vi "SendThread.vi"() -> ()   [LabVIEW 2011]
uses:
  VIs/_USB_CAN_T_R_Unit_.ctl
  VIs/_USB_CAN_GLOBAL_.vi
panel:
  in  "channels":i32=2
  in  "TFun":u16
  in  "DeviceInd":u32
  in  "channel":u16(ring) items=["通道0", "通道1"]
  in  "type":u16(ring)=2 items=["USB-CAN"=2, "USB-CAN2.0"=3]
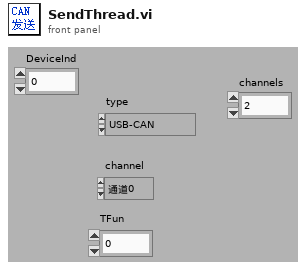
[diagram p1: front panel]
types:
  T1 = typedef "_USB_CAN_T_R_Unit_.ctl" = cluster{"time":timestamp, "channel":u16, "TimeStamp":u32, "tr":enum16{"接收", "发送"}, "id":u32, "Type":enum16{"数据帧", "远程帧"}, "Format":enum16{"标准帧", "扩展帧"}, "len":u8, "data":u8[]}
  T2 = typedef "_USB_CAN_SEND_BUFF_UNIT_.ctl" = cluster{"datalen":u8, "data":u8[], "id":u8[], "extended":bool, "remote":bool}
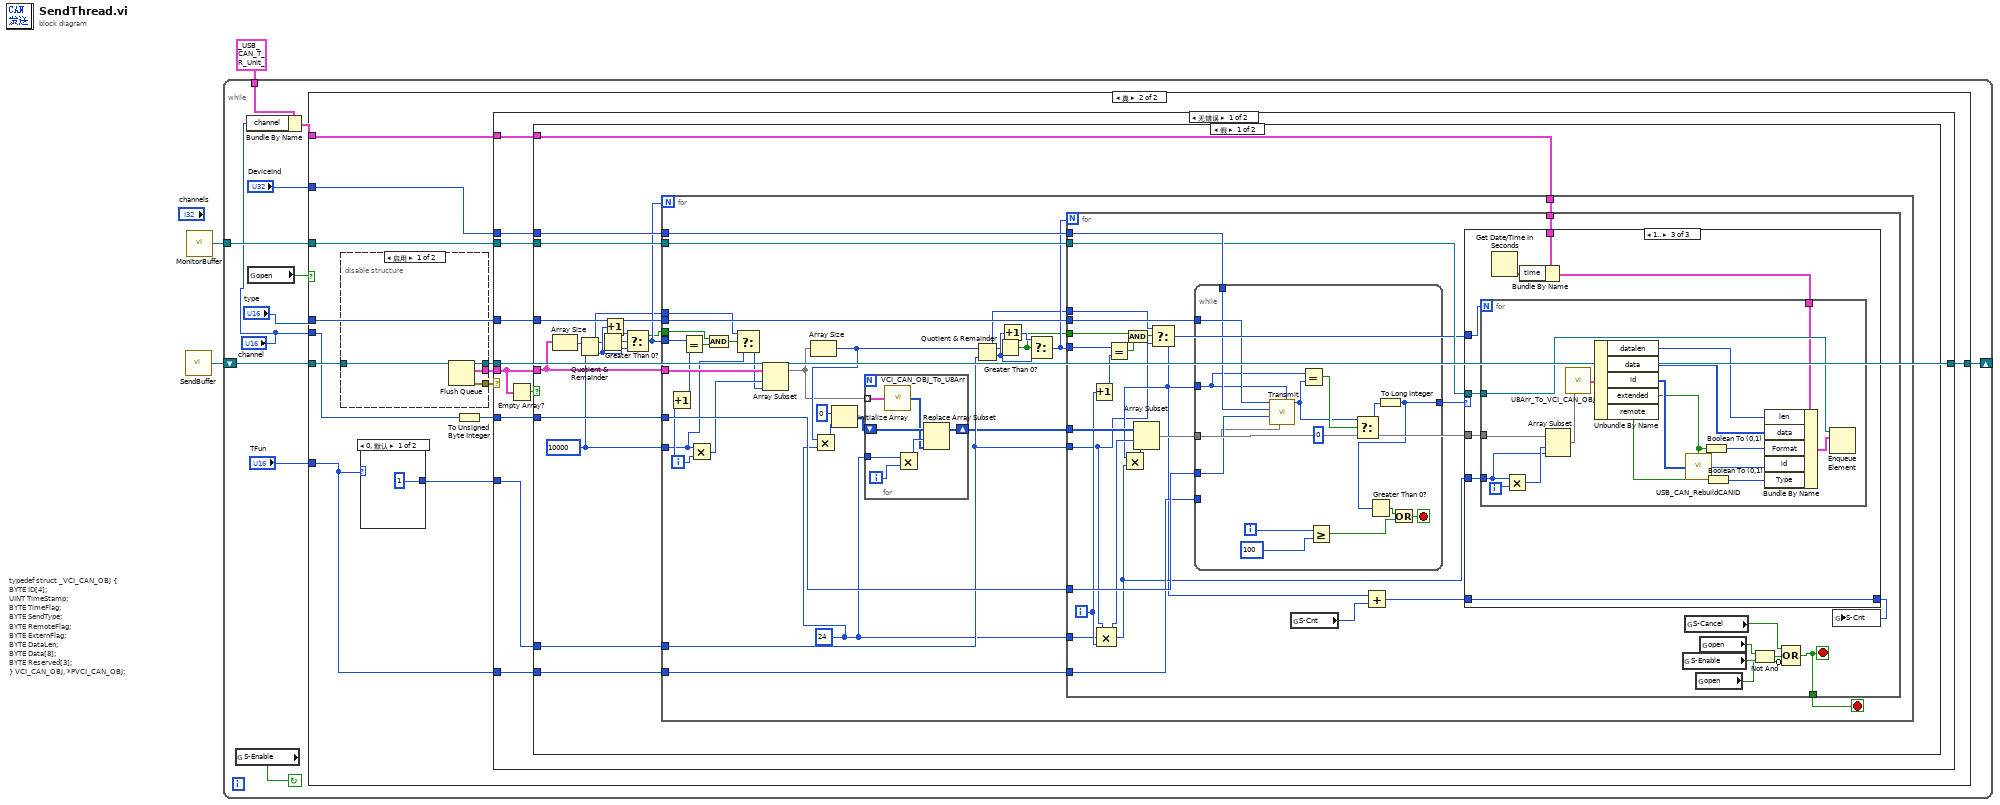
[diagram p0: block diagram]
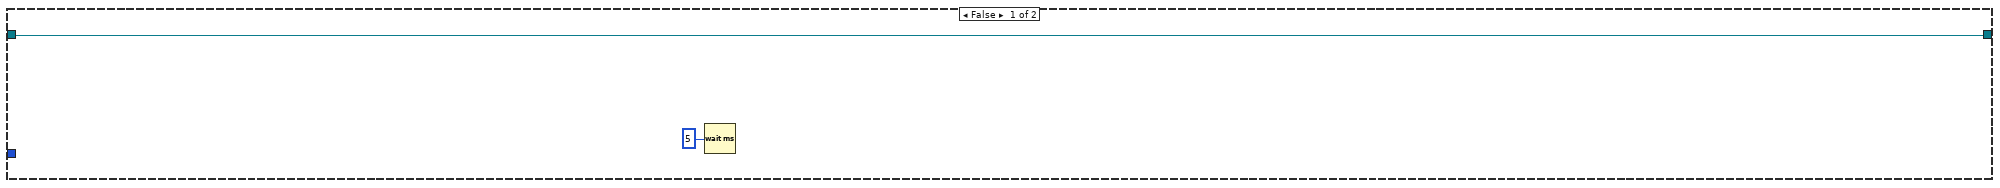
[diagram p2: hidden frame]
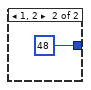
[diagram p3: hidden frame]
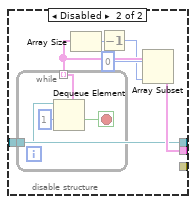
[diagram p4: hidden frame]
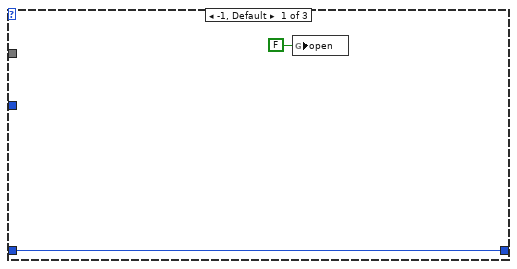
[diagram p5: hidden frame]
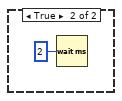
[diagram p7: hidden frame]
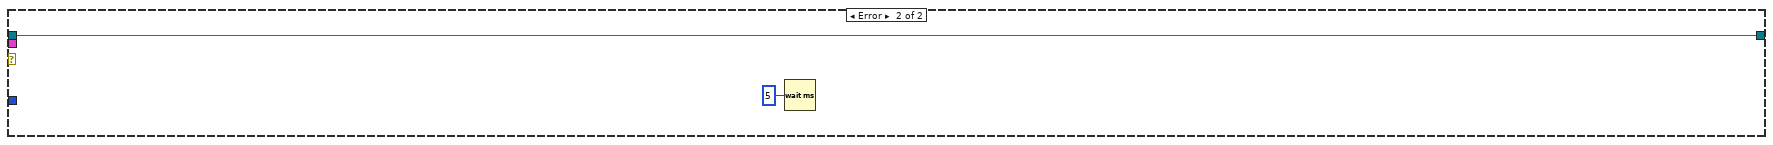
[diagram p8: hidden frame]
diagram:
  # "typedef struct _VCI_CAN_OBJ { \nBYTE ID[4];\nUINT TimeStamp; \nBYTE TimeFlag;\nBYTE SendType; \nBYTE RemoteFlag; \nBYTE ExternFlag; \nBYTE DataLen; \nBYTE Data[8]; \nBYTE Reserved[3];\n} VCI_CAN_OBJ, *PVCI_CAN_OBJ;"
  n1 = call "SendBuffer.vi"() -> ("VCI_CAN_BUF_T"=w3:refnum<queue>)  [unwired: 1 in]
  n2 = call "MonitorBuffer.vi"() -> ("USB_CAN_M_BUF"=w2:refnum<queue>)  [unwired: 1 in]
  n3 = while {
    shift-right: [w13] -> _
    shift-left: w3 -> [w14]
    tunnel: w2 -> [w8]
    tunnel: T1 {"time"=timestamp(0 s since 1904-01-01), "channel"=0, "TimeStamp"=0, "tr"=enum."发送", "id"=0, "Type"=enum."数据帧", "Format"=enum."标准帧", "len"=0, "data"=[]} ("元素") -> [w7]
    stop <- w12 continue-if-true
    n4 = global read "_USB_CAN_GLOBAL_.vi" "S-Enable"() -> (w12:bool)
    n5 = Bundle By Name(cluster=w7, "channel"="channel") -> (w5:T1)
    n6 = global read "_USB_CAN_GLOBAL_.vi" "open"() -> (w11:bool)
    n7 = case shown="真" w11 {
      tunnel: "type" -> [_ w25]
      tunnel: "channel" -> [_ w24]
      tunnel: w14 -> [w16 w29]
      tunnel: [w16 w26] -> w13
      tunnel: w8 -> [_ w22]
      tunnel: "DeviceInd" -> [_ w21]
      tunnel: "TFun" -> [_ w18]
      tunnel: w5 -> [_ w19]
      frame False {
        n8 = Wait (ms)(milliseconds to wait=u32 5 ("millisecond multiple")) -> ()  [unwired: 1 out]
      }
      frame True {
        n9 = disable-structure shown="启用" {
          disable-tunnel: w29 -> [w35 w36]
          disable-tunnel: [w34 _] -> w28
          disable-tunnel: [w33 w36] -> w27
          disable-tunnel: [w32 w37] -> w20
          frame Enabled {
            n10 = Flush Queue(queue=w35) -> (queue out=w33:refnum<queue>, remaining elements=w32:T2[], error out=w34:errorcluster)  [unwired: 1 in]
          }
          frame Disabled {
            n11 = while {
              tunnel: w36 -> [w45]
              tunnel: [w43] -> w40 mode=indexing
              stop <- w42 stop-if-true
              n12 = Dequeue Element(queue=w45, timeout in ms (-1)=1 ("超时毫秒(-1)")) -> (element=w43:T2, timed out?=w42:bool)  [unwired: 1 in, 2 out]
            }
            n13 = Array Size(array=w40) -> (size(s)=w41:i32)
            n14 = Decrement(x=w41) -> (x-1=w38:i32)
            n15 = Array Subset(array=w40, index=0 ("索引"), length=w38) -> (w37:T2[])
          }
        }
        n16 = case shown="0, 默认" w18 {
          tunnel: [1 ("索引") 48 ("索引")] -> w17
          frame 0, Default {
          }
          frame 1, 2 {
          }
        }
        n17 = To Unsigned Byte Integer(number=w24) -> (unsigned 8bit integer=w23:u8)
        n18 = case shown="无错误" w28 {
          tunnel: w27 -> [w50 w184]
          tunnel: [w50 w184] -> w26
          tunnel: w20 -> [w48 _]
          tunnel: w25 -> [w51 _]
          tunnel: w23 -> [w54 _]
          tunnel: w22 -> [w49 _]
          tunnel: w21 -> [w55 _]
          tunnel: w17 -> [w53 _]
          tunnel: w18 -> [w52 _]
          tunnel: w19 -> [w46 _]
          frame No Error {
            n19 = Empty Array?(array=w48) -> (empty?=w47:bool)
            n20 = case shown="假" w47 {
              tunnel: w55 -> [w70 _]
              tunnel: w54 -> [w69 _]
              tunnel: w53 -> [w65 _]
              tunnel: w52 -> [w68 _]
              tunnel: w51 -> [w67 _]
              tunnel: w49 -> [w66 _]
              tunnel: w48 -> [w63 _]
              tunnel: w46 -> [w64 _]
              frame False {
                w59 = 10000 ("y")
                n21 = Array Size(array=w63) -> (size(s)=w62:i32)
                n22 = Quotient & Remainder(x=w62, y=w59) -> (x-y*floor(x/y)=w56:i32, floor(x/y)=w60:i32)
                n23 = Greater Than 0?(x=w56) -> (x > 0?=w57:bool)
                n24 = Increment(x=w60) -> (x+1=w61:i32)
                n25 = Select(t=w61, s=w57, f=w60) -> (s? t:f=w58:i32)
                n26 = for {
                  N: w58 -> [_]
                  tunnel: w70 -> [w101]
                  tunnel: w69 -> [w100]
                  tunnel: w68 -> [w99]
                  tunnel: w67 -> [w98]
                  tunnel: w66 -> [w97]
                  tunnel: w65 -> [w96]
                  tunnel: w64 -> [w95]
                  tunnel: w63 -> [w83]
                  tunnel: w59 -> [w73]
                  tunnel: w58 -> [w79]
                  tunnel: w57 -> [w76]
                  tunnel: w56 -> [w74]
                  i -> [w80]
                  stop <- w71 stop-if-true
                  w86 = 24 ("x")
                  n27 = Increment(x=w80) -> (x+1=w78:i32)
                  n28 = Equal?(x=w79, y=w78) -> (x = y?=w77:bool)
                  n29 = Multiply(x=w73, y=w80) -> (x*y=w81:i32)
                  n30 = And(x=w76, y=w77) -> (x .and. y?=w75:bool)
                  n31 = Select(t=w74, s=w75, f=w73) -> (s? t:f=w72:i32)
                  n32 = Array Subset(array=w83, index=w81, length=w72) -> (w82:T2[])
                  n33 = Array Size(array=w82) -> (size(s)=w84:i32)
                  n34 = Multiply(x=w84, y=w86) -> (x*y=w87:i32)
                  n35 = Initialize Array(u8 0, w87) -> (w85:u8[])
                  n36 = for {
                    tunnel: w82 -> [w176] mode=indexing
                    shift-right: [w181] -> w94
                    shift-left: w85 -> [w180]
                    tunnel: w86 -> [w177]
                    i -> [w179]
                    n37 = call "VCI_CAN_OBJ_To_U8Arr.vi"("VCI_CAN_BUF_T"=w176) -> ("U8 Arr"=w175:u8[])
                    n38 = Multiply(x=w177, y=w179) -> (x*y=w178:i32)
                    n39 = Replace Array Subset(array=w180, new element=w175, index=w178) -> (w181:u8[])
                  }
                  n40 = Quotient & Remainder(x=w84, y=w96) -> (x-y*floor(x/y)=w89:i32, floor(x/y)=w93:i32)
                  n41 = Greater Than 0?(x=w89) -> (x > 0?=w90:bool)
                  n42 = Increment(x=w93) -> (x+1=w92:i32)
                  n43 = Select(t=w92, s=w90, f=w93) -> (s? t:f=w91:i32)
                  n44 = for {
                    N: w91 -> [_]
                    tunnel: w101 -> [w131]
                    tunnel: w100 -> [w130]
                    tunnel: w99 -> [w129]
                    tunnel: w98 -> [w128]
                    tunnel: w97 -> [w127]
                    tunnel: w94 -> [w125]
                    tunnel: w86 -> [w107]
                    tunnel: w96 -> [w102]
                    tunnel: w91 -> [w122]
                    tunnel: w90 -> [w121]
                    tunnel: w89 -> [w118]
                    tunnel: w95 -> [w115]
                    tunnel: [w103] -> w71
                    i -> [w124]
                    stop <- w103 stop-if-true
                    n45 = Increment(x=w124) -> (x+1=w123:i32)
                    n46 = Compound Arithmetic op=MULTIPLY(w102, w107, w124) -> (w106:i32)
                    n47 = Equal?(x=w122, y=w123) -> (x = y?=w120:bool)
                    n48 = And(x=w121, y=w120) -> (x .and. y?=w119:bool)
                    n49 = Select(t=w118, s=w119, f=w102) -> (s? t:f=w105:i32)
                    n50 = Multiply(x=w105, y=w107) -> (x*y=w116:i32)
                    n51 = Array Subset(array=w125, index=w106, length=w116) -> (w117:u8[])
                    n52 = while {
                      tunnel: w131 -> [w139]
                      tunnel: w130 -> [w146]
                      tunnel: w129 -> [_]
                      tunnel: w128 -> [w145]
                      tunnel: [w132] -> w126
                      tunnel: w117 -> [w144]
                      tunnel: w105 -> [w134]
                      i -> [w143]
                      stop <- w140 stop-if-true
                      n53 = call "Transmit.vi"("Len"=w134, "pSend"=w144, "CANInd"=w146, "DeviceInd"=w139, "type"=w145) -> ("Success"=w135:u32)  [unwired: 5 in, 1 out]
                      n54 = Equal?(x=w134, y=w135) -> (x = y?=w138:bool)
                      n55 = Greater Or Equal?(x=w143, y=100) -> (x >= y?=w141:bool)
                      n56 = Select(t=w135, s=w138, f=u32 0) -> (s? t:f=w133:u32)
                      n57 = To Long Integer(number=w133) -> (32bit integer=w132:i32)
                      n58 = Greater Than 0?(x=w132) -> (x > 0?=w136:bool)
                      n59 = Or(x=w136, y=w141) -> (x .or. y?=w140:bool)
                    }
                    n60 = global read "_USB_CAN_GLOBAL_.vi" "S-Cnt"() -> (w110:i64)
                    n61 = Add(x=w105, y=w110) -> (x+y=w109:i64)
                    n62 = case shown="1.." w126 {
                      tunnel: w127 -> [_ _ w157]
                      tunnel: w105 -> [_ _ w156]
                      tunnel: w117 -> [_ _ w155]
                      tunnel: w115 -> [_ _ w153]
                      tunnel: w109 -> [w148 w149 w151]
                      tunnel: [w148 w149 w151] -> w108
                      tunnel: w107 -> [_ _ w150]
                      frame -1, Default {
                        n63 = global write "_USB_CAN_GLOBAL_.vi" "open"(FALSE ("open")) -> ()
                      }
                      frame 0 {
                      }
                      frame 1.. {
                        n64 = Get Date/Time In Seconds() -> (seconds since 1Jan1904=w154:timestamp)
                        n65 = Bundle By Name(cluster=w153, "time"=w154) -> (w152:T1)
                        n66 = for {
                          N: w156 -> [_]
                          tunnel: w157 -> [w174]
                          tunnel: w155 -> [w162]
                          tunnel: w152 -> [w173]
                          tunnel: w150 -> [w159]
                          i -> [w161]
                          n67 = Multiply(x=w159, y=w161) -> (x*y=w160:i32)
                          n68 = Array Subset(array=w162, index=w160, length=w159) -> (w158:u8[])
                          n69 = call "U8Arr_To_VCI_CAN_OBJ.vi"("U8 Arr"=w158) -> ("VCI_CAN_BUF_T"=w172:T2)
                          n70 = Unbundle By Name(w172) -> ("datalen"=w165:u8, "data"=w164:u8[], "id"=w170:u8[], "extended"=w166:bool, "remote"=w168:bool)
                          n71 = call "USB_CAN_RebuildCANID.vi"("ExtFrame"=w166, "IDS"=w170) -> ("ID"=w171:u32)  [unwired: 2 in]
                          n72 = Boolean To (0,1)(Boolean=w166) -> (0, 1=w167:i16)
                          n73 = Boolean To (0,1)(Boolean=w168) -> (0, 1=w169:i16)
                          n74 = Bundle By Name(cluster=w173, "len"=w165, "data"=w164, "Format"=w167, "id"=w171, "Type"=w169) -> (w163:T1)
                          n75 = Enqueue Element(queue=w174, element=w163) -> ()  [unwired: 2 in, 3 out]
                        }
                      }
                    }
                    n76 = global read "_USB_CAN_GLOBAL_.vi" "S-Enable"() -> (w113:bool)
                    n77 = global read "_USB_CAN_GLOBAL_.vi" "S-Cancel"() -> (w111:bool)
                    n78 = global read "_USB_CAN_GLOBAL_.vi" "open"() -> (w104:bool)
                    n79 = global read "_USB_CAN_GLOBAL_.vi" "open"() -> (w114:bool)
                    n80 = Not And(1:w113, 2:w114) -> (0:w112:bool)
                    n81 = Compound Arithmetic op=OR(w111, w112, invert w104) -> (w103:bool)
                    n82 = global write "_USB_CAN_GLOBAL_.vi" "S-Cnt"(w108) -> ()
                  }
                }
              }
              frame True {
                n83 = Wait (ms)(milliseconds to wait=u32 2 ("等待时间（毫秒）")) -> ()  [unwired: 1 out]
              }
            }
          }
          frame Error {
            n84 = Wait (ms)(milliseconds to wait=u32 5 ("等待时间（毫秒）")) -> ()  [unwired: 1 out]
          }
        }
      }
    }
  }
